vi "G#Object_ExternalCreateProcessDelegate.vi"(0 "delegate event out":refnum<user-event>, 1 "event queue":refnum<queue>, 5 "error in (no error)":errorcluster) -> (19 "error out":errorcluster)   [LabVIEW 2020, in "G#Object.lvclass"]
doc: "This is a delegate process that creates the object specified by the events."
uses:
  G#Object.lvclass
  utils/G#Object_Event.ctl
  utils/G#Object_EventType.ctl
  utils/G#Object_ObjectInfoType.ctl
  utils/G#Object_CreateMethod.ctl
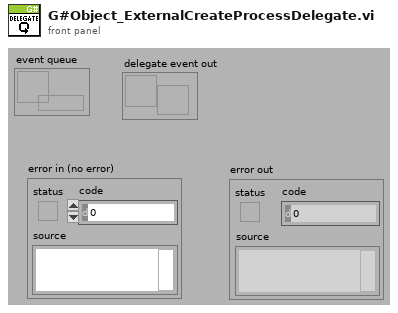
[diagram p1: front panel]
types:
  T1 = typedef "G#Object.lvclass/G#Object_EventType.ctl" = enum16{"Created new", "Looked up existing", "Deleted", "Forced delete", "Not deleted", "Garbage collected", "Cleared", "User", "Error", "External create object", "External create class attributes", "Created class attributes", "Run constructor", "Run constructor done", "Run open method", "Run open method done"}
  T2 = typedef "G#Object.lvclass/G#Object_ObjectInfoType.ctl" = cluster{"ObjectName":string, "ObjectID":u32, "Users":i32, "Counter":bool, "AttributeRefs":u32[], "FullClassName":string, "ClassName":string, "CreateMethod":T3, "GenericDestructorExists":bool, "Owner":string}
  T3 = typedef "G#Object.lvclass/G#Object_CreateMethod.ctl" = enum16{"Create", "Create or look up existing", "Look up existing"}
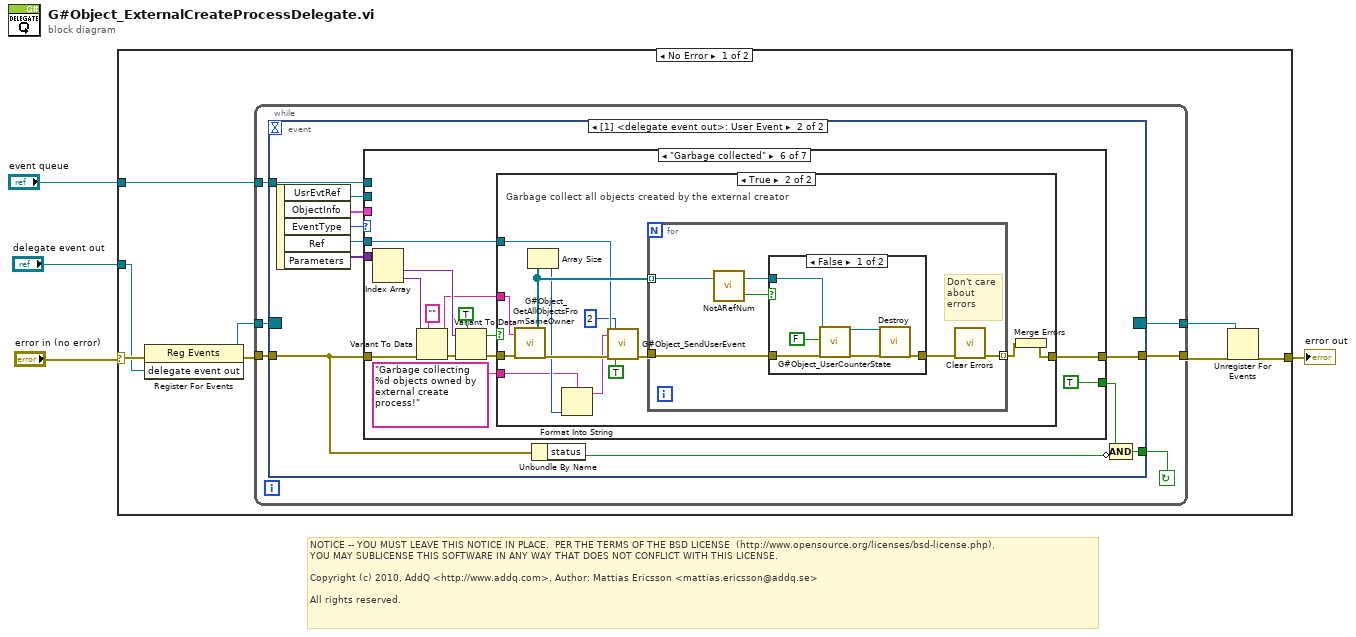
[diagram p0: block diagram]
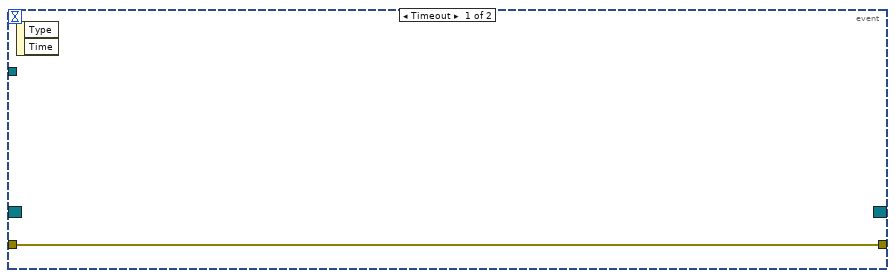
[diagram p2: hidden frame]
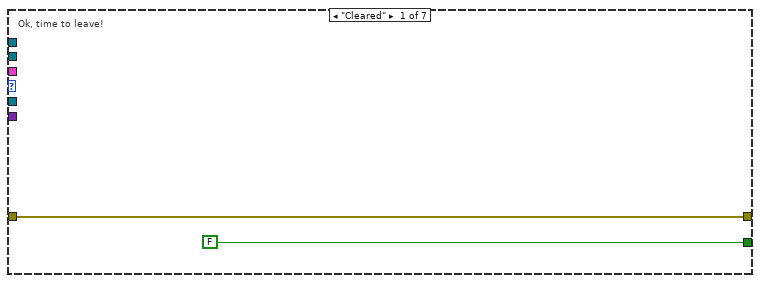
[diagram p3: hidden frame]
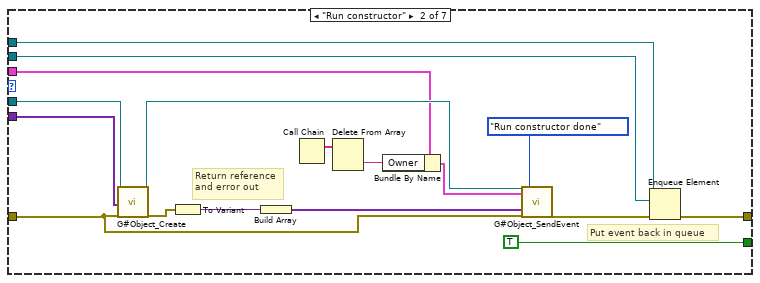
[diagram p4: hidden frame]
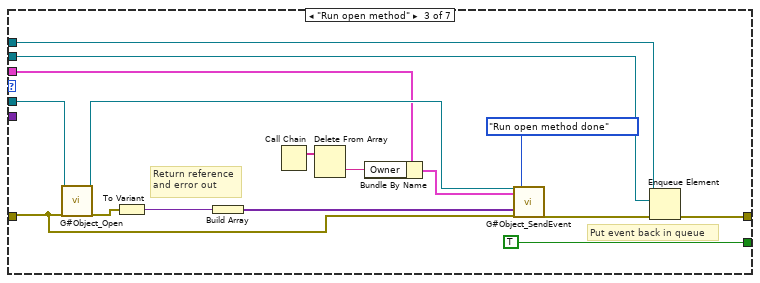
[diagram p5: hidden frame]
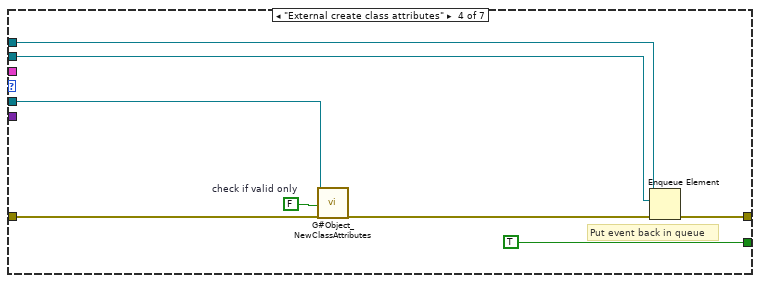
[diagram p6: hidden frame]
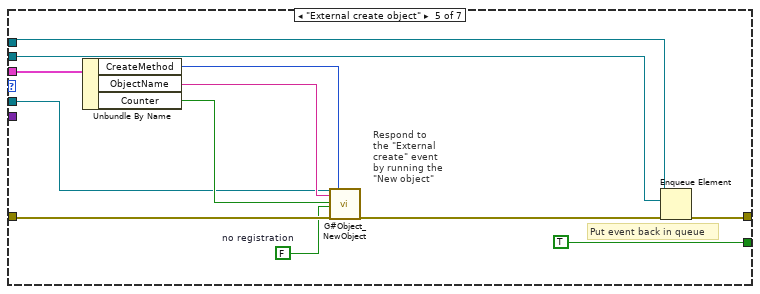
[diagram p7: hidden frame]
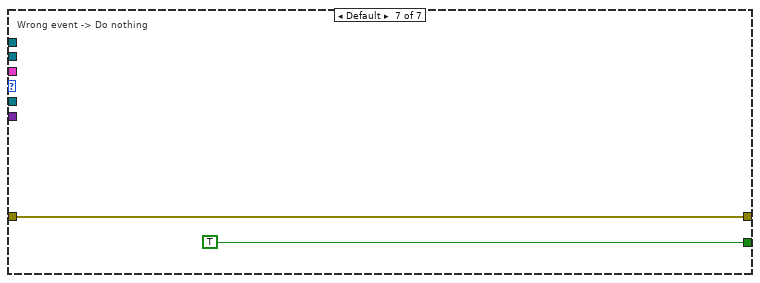
[diagram p10: hidden frame]
diagram:
  # "NOTICE -- YOU MUST LEAVE THIS NOTICE IN PLACE.  PER THE TERMS OF THE BSD LICENSE  (http://www.opensource.org/licenses/bsd-license.php).\nYOU MAY SUBLICENSE THIS SOFTWARE IN ANY WAY THAT DOES NOT CONFLICT WITH THIS LICENSE.\n\nCopyright (c) 2010, AddQ <http://www.addq.com>, Author: Mattias Ericsson <mattias.ericsson@addq.se>\n\nAll rights reserved."
  n1 = case shown="No Error" "error in (no error)" {
    selector: "error in (no error)" -> [w9 w129]
    tunnel: [w11 w129] -> w4
    tunnel: "event queue" -> [w12 _]
    tunnel: "delegate event out" -> [w8 _]
    frame No Error {
      n2 = register-events(error in=w9, w8) -> (reference out=w6:refnum<event-registration>, error out=w7:errorcluster)  [unwired: 1 in]
      n3 = while {
        tunnel: w7 -> [w18]
        tunnel: [w17] -> w10
        tunnel: w12 -> [w15]
        tunnel: w6 -> [w14]
        tunnel: [w13] -> w5
        stop <- w16 continue-if-true
        n4 = event shown="[1] <delegate event out>: User Event" {
          selector: w14 -> [_ _]
          dyn-events: [_ _] -> w13
          timeout: _ -> [_ _]
          tunnel: w18 -> [w19 w28]
          tunnel: [w19 w30] -> w17
          tunnel: [_ w25] -> w16
          tunnel: w15 -> [_ w22]
          event Timeout {
            n5 = event-data() -> ()  [unwired: 1 in, 2 out]
          }
          event User Event {
            n6 = event-data() -> ("UsrEvtRef"=w21:refnum<user-event>, "ObjectInfo"=w23:T2, "EventType"=w29:T1, "Ref"=w20:refnum<class "G#Object.lvclass">, "Parameters"=w24:variant[])  [unwired: 1 in]
            n7 = case shown="\"Garbage collected\"" w29 {
              tunnel: w28 -> [w32 w38 w55 w68 w81 w96 w127]
              tunnel: [w32 w44 w60 w72 w78 w98 w127] -> w30
              tunnel: [FALSE TRUE TRUE TRUE TRUE TRUE TRUE] -> w26
              tunnel: w24 -> [_ w33 _ _ _ w99 _]
              tunnel: w23 -> [_ w37 w51 _ w82 _ _]
              tunnel: w22 -> [_ w43 w59 w71 w77 _ _]
              tunnel: w21 -> [_ w42 w58 w70 w76 _ _]
              tunnel: w20 -> [_ w41 w57 w69 w75 w87 _]
              frame "Cleared" {
                # "Ok, time to leave!"
              }
              frame "Run constructor" {
                # "Put event back in queue"
                # "Return reference\nand error out"
                n8 = call-dynamic "G#Object_Create.vi"("reference in"=w41, "control values"=w33, "error in (no error)"=w38) -> ("reference out"=w40:refnum<class "G#Object.lvclass">, "error out"=w48:errorcluster)  [unwired: 15 in]
                n9 = To Variant(anything=w48) -> (Variant=w47:variant)
                n10 = Build Array(w47) -> (w45:variant[])
                n11 = Call Chain() -> (call chain=w35:string[])
                n12 = Delete From Array(array=w35) -> (deleted portion=w34:string)  [unwired: 2 in, 1 out]
                n13 = Bundle By Name(cluster=w37, "Owner"=w34) -> (w36:T2)
                n14 = call "G#Object_SendEvent.vi"("reference in"=w40, "object info extended"=w36, "parameters"=w45, "error in (no error)"=w38, "G# event type"=G#Object_EventType."Run constructor done") -> ("error out"=w39:errorcluster)  [unwired: 14 in]
                n15 = Enqueue Element(queue=w43, element=w42, error in (no error)=w39) -> (error out=w44:errorcluster)  [unwired: 1 in, 2 out]
              }
              frame "Run open method" {
                # "Put event back in queue"
                # "Return reference\nand error out"
                n16 = call-dynamic "G#Object_Open.vi"("reference in"=w57, "error in (no error)"=w55) -> ("reference out"=w56:refnum<class "G#Object.lvclass">, "error out"=w64:errorcluster)  [unwired: 16 in]
                n17 = To Variant(anything=w64) -> (Variant=w63:variant)
                n18 = Build Array(w63) -> (w61:variant[])
                n19 = Call Chain() -> (call chain=w53:string[])
                n20 = Delete From Array(array=w53) -> (deleted portion=w52:string)  [unwired: 2 in, 1 out]
                n21 = Bundle By Name(cluster=w51, "Owner"=w52) -> (w50:T2)
                n22 = call "G#Object_SendEvent.vi"("reference in"=w56, "object info extended"=w50, "parameters"=w61, "error in (no error)"=w55, "G# event type"=G#Object_EventType."Run open method done") -> ("error out"=w54:errorcluster)  [unwired: 14 in]
                n23 = Enqueue Element(queue=w59, element=w58, error in (no error)=w54) -> (error out=w60:errorcluster)  [unwired: 1 in, 2 out]
              }
              frame "External create class attributes" {
                w66 = FALSE  # check if valid only
                # "Put event back in queue"
                n24 = call "G#Object_NewClassAttributes.vi"("reference in"=w69, "check if valid only (F)"=w66, "error in (no error)"=w68) -> ("error out"=w67:errorcluster)  [unwired: 12 in, 4 out]
                n25 = Enqueue Element(queue=w71, element=w70, error in (no error)=w67) -> (error out=w72:errorcluster)  [unwired: 1 in, 2 out]
              }
              frame "External create object" {
                w74 = FALSE  # no registration
                # "Put event back in queue"
                # "Respond to\nthe \"External\ncreate\" event\nby running the\n\"New object\""
                n26 = Unbundle By Name(w82) -> ("CreateMethod"=w85:T3, "ObjectName"=w84:string, "Counter"=w83:bool)
                n27 = call "G#Object_NewObject.vi"("reference in"=w75, "object name (\"\")"=w84, "user counter (T)"=w83, "no registration (F)"=w74, "error in (no error)"=w81, "create method"=w85) -> ("error out"=w79:errorcluster)  [unwired: 11 in, 2 out]
                n28 = Enqueue Element(queue=w77, element=w76, error in (no error)=w79) -> (error out=w78:errorcluster)  [unwired: 1 in, 2 out]
              }
              frame "Garbage collected" {
                n29 = Index Array(array=w99) -> (element #1=w92:variant, element #2=w93:variant)  [unwired: 2 in]
                n30 = Variant To Data(error in=w96, type="", Variant=w93) -> (data=w88:string, error out=w95:errorcluster)
                n31 = Variant To Data(error in=w95, type=TRUE, Variant=w92) -> (data=w89:bool, error out=w94:errorcluster)
                n32 = case shown="True" w89 {
                  tunnel: [w100 w113] -> w98
                  tunnel: w94 -> [w100 w111]
                  tunnel: w88 -> [_ w110]
                  tunnel: w87 -> [_ w106]
                  tunnel: "Garbage collecting %d objects owned by external create process!" -> [_ w103]
                  frame False {
                  }
                  frame True {
                    # "Garbage collect all objects created by the external creator"
                    n33 = call "G#Object_GetAllObjectsFromSameOwner.vi"("full class name (\"\")"=w110, "error in (no error)"=w111) -> ("all refs"=w109:refnum<class "G#Object.lvclass">[], "error out"=w108:errorcluster)  [unwired: 14 in, 2 out]
                    n34 = Array Size(array=w109) -> (size(s)=w105:i32)
                    n35 = Format Into String(format string=w103, w105) -> (resulting string=w104:string)  [unwired: 2 in, 1 out]
                    n36 = call "G#Object_SendUserEvent.vi"("refererence in"=w106, "text"=w104, "error in (no error)"=w108, "call depth (1)"=2 ("call depth"), "send to Desktop Trace Execution? (F)"=TRUE ("send to Desktop Trace Execution")) -> ("error out"=w107:errorcluster)  [unwired: 13 in, 1 out]
                    n37 = for {
                      tunnel: w107 -> [w114]
                      tunnel: [w118] -> w112 mode=indexing
                      tunnel: w109 -> [w117] mode=indexing
                      # "Don't care\nabout\nerrors"
                      n38 = call-dynamic "NotARefNum.vi"("reference in"=w117) -> ("not a refnum?"=w116:bool, "reference out"=w115:refnum<class "G#Object.lvclass">)  [unwired: 1 in]
                      n39 = case shown="False" w116 {
                        tunnel: [w125 w126] -> w119
                        tunnel: w114 -> [w124 w126]
                        tunnel: w115 -> [w122 _]
                        frame False {
                          n40 = call "G#Object_UserCounterState.vi"("reference in"=w122, "user counter (F)"=FALSE, "error in (no error)"=w124) -> ("reference out"=w120:refnum<class "G#Object.lvclass">, "error out"=w123:errorcluster)  [unwired: 15 in]
                          n41 = call-dynamic "Destroy.vi"("reference in"=w120, "error in (no error)"=w123) -> ("error out"=w125:errorcluster)  [unwired: 16 in, 1 out]
                        }
                        frame True {
                        }
                      }
                      n42 = call <vilib>:"Clear Errors.vi"("error in (no error)"=w119) -> ("error out"=w118:errorcluster)  [unwired: 5 in, 1 out]
                    }
                    n43 = Merge Errors(w112) -> (w113:errorcluster)
                  }
                }
              }
              frame Default {
                # "Wrong event -> Do nothing"
              }
            }
            n44 = Unbundle By Name(w28) -> ("status"=w27:bool)
            n45 = Compound Arithmetic op=AND(w26, invert w27) -> (w25:bool)
          }
        }
      }
      n46 = Unregister For Events(event registration refnum=w5, error in=w10) -> (error out=w11:errorcluster)
    }
    frame Error {
    }
  }
  "error out" <- w4
